vi "Call.vi"(7 "Class Instance":T1, 8 "error in (no error)":errorcluster, 9 "Arguments":T1[](array[typedef]), 10 "Function/Method Name":string, 11 "Session Handle in":refnum<data-value>) -> (0 "error out":errorcluster, 1 "Returned Python Object Refnum":T1, 3 "Session Handle out":refnum<data-value>)   [LabVIEW 2020, in "G-Embedded-Python-Interpreter-Toolkit.lvlib"]
uses:
  G-Embedded-Python-Interpreter-Toolkit.lvlib
  Python Object Reference.ctl
  Python Object Type.ctl
  bin/gepit.cp310.32.dll
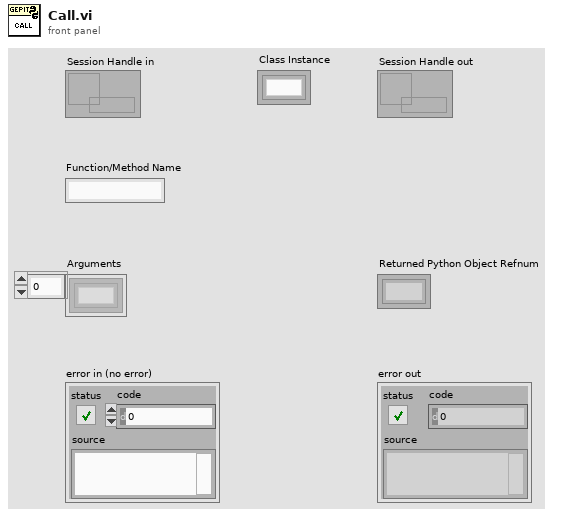
[diagram p1: front panel]
types:
  T1 = typedef "G-Embedded-Python-Interpreter-Toolkit.lvlib/Python Object Reference.ctl" = refnum<k1>
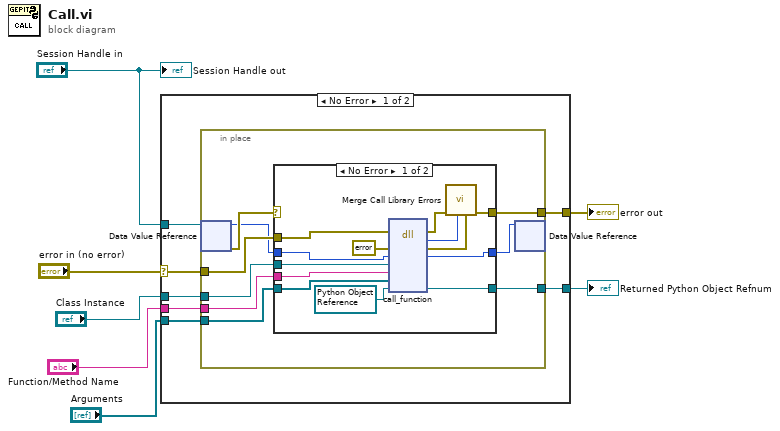
[diagram p0: block diagram]
diagram:
  n1 = case shown="No Error" "error in (no error)" {
    selector: "error in (no error)" -> [w13 w39]
    tunnel: "Session Handle in" -> [w14 _]
    tunnel: [w12 w39] -> w6
    tunnel: "Arguments" -> [w11 _]
    tunnel: [w10 _] -> w2
    tunnel: "Function/Method Name" -> [w9 _]
    tunnel: "Class Instance" -> [w8 _]
    frame No Error {
      n2 = in-place {
        in-place-border: w13 -> [w22]
        in-place-border: [w19] -> w12
        in-place-border: w11 -> [w18]
        in-place-border: [w17] -> w10
        in-place-border: w9 -> [w16]
        in-place-border: w8 -> [w15]
        n3 = in-place-dvr #1(w14) -> (w21:u64, w23:errorcluster)
        n4 = case shown="No Error" w23 {
          selector: w23 -> [_ w37]
          tunnel: w22 -> [w32 _]
          tunnel: w21 -> [w31 w38]
          tunnel: [w30 w38] -> w20
          tunnel: [w29 w37] -> w19
          tunnel: w18 -> [w26 _]
          tunnel: [w28 _] -> w17
          tunnel: w16 -> [w25 _]
          tunnel: w15 -> [w24 _]
          frame No Error {
            w27 = T1 refnum items=["PObj"] ("Returned Python Object Refnum")
            n5 = dll-call lib="C:/serenial/libraries/g-embedded-python-interpreter-toolkit/LabVIEW/bin/gepit.cp310.32.dll" fn="call_function"(error in=w32, "Error"=errorcluster {"status"=FALSE, "code"=0, "source"=""} ("error constant"), "Session"=w31, "Class Instance"=w24, "Function Name"=w25, "Arguments"=w26, "Return"=w27) -> (error out=w35:errorcluster, "return type"=w34:i32, "Error"=w33:errorcluster, "Session"=w30:u64, "Return"=w28:T1)  [unwired: 5 in, 1 out]
            n6 = call "Merge Call Library Errors.vi"("Call Library Error"=w33, "Return Value"=w34, "error in"=w35) -> ("error out"=w29:errorcluster)  [unwired: 8 in]
          }
          frame Error {
          }
        }
        n7 = in-place-dvr #1(w20) -> ()  [unwired: 2 out]
      }
    }
    frame Error {
    }
  }
  "error out" <- w6
  "Returned Python Object Refnum" <- w2
  "Session Handle out" <- "Session Handle in"
